vi "Continuous Pulse Train Test (IPD).vi"() -> ()   [LabVIEW 2015]
uses:
  Waveform VIs/Pulse Train VIs/Pulse Train Params.ctl
  Waveform VIs/Pulse Train VIs/Pulse Polarity.ctl
  Waveform VIs/Pulse Train VIs/PT-Continuous State.ctl
  <vilib>/sound2/lvsound2.llb/Sound Data Format.ctl
  <vilib>/sound2/lvsound2.llb/Sampling Mode.ctl
  <vilib>/sound2/lvsound2.llb/Sound Output Write (DBL).vi
panel:
  in  "IPD (cycles)":dbl(slide)=0.5 min=-0.5 max=0.5 scale=-0.5..0.5
  in  "stop":bool
  in  "Sound Format":T1={"sample rate (S/s)"=50000.0, "number of channels"=2, "bits per sample"=16}
  in  "Device ID":u32
  in  "Pulse Train Params":T2={"Pulse width (us)"=100.0, "Pulse rate (Hz)"=0.0, "Gap (ms)"=0.0, "Polarity"=enum."NEG-POS", "PT State"={"Template"=[], "Nperiod"=0, "Index"=0, "Pulse Rate (Hz)"=0.0, "Phase (cycles)"=0.0, "Noff"=0}, "Asynch"=FALSE}
  out "Graph":waveform(dbl)[](graph)
  in  "Buffer (ms)":dbl=100.0
  in  "Pulse Rate (Hz)":dbl(slide)=36.55555555555556 min=1.0 max=100.0 scale=1.0..100.0
  in  "Fs (Hz)":dbl=100000.0
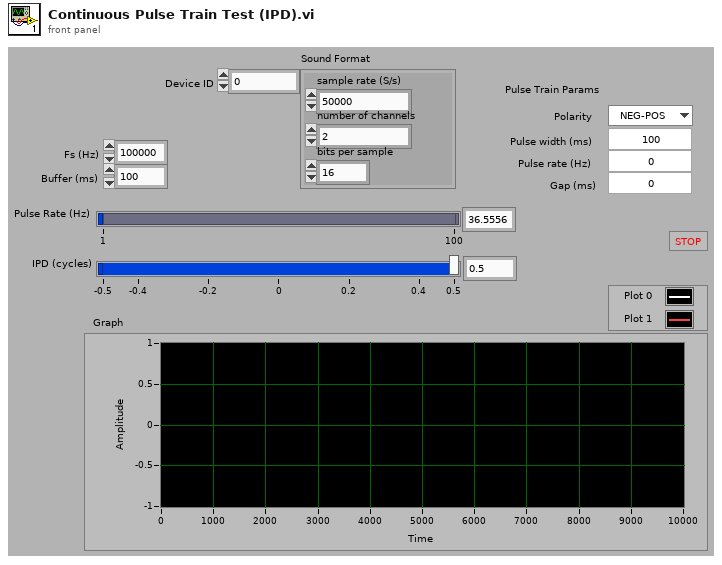
[diagram p1: front panel]
types:
  T1 = typedef "Sound Data Format.ctl" = cluster{"sample rate (S/s)":dbl, "number of channels":i32, "bits per sample":i32}
  T2 = typedef "Pulse Train Params.ctl" = cluster{"Pulse width (us)":dbl, "Pulse rate (Hz)":dbl, "Gap (ms)":dbl, "Polarity":T3, "PT State":T4, "Asynch":bool}
  T3 = typedef "Pulse Polarity.ctl" = enum16{"POS", "NEG", "POS-NEG", "NEG-POS"}
  T4 = typedef "PT-Continuous State.ctl" = cluster{"Template":dbl[], "Nperiod":i32, "Index":i32, "Pulse Rate (Hz)":dbl, "Phase (cycles)":dbl, "Noff":i32}
  T5 = typedef "Sampling Mode.ctl" = i32
  T6 = typedef "Sound Output Task ID.ctl" = u32
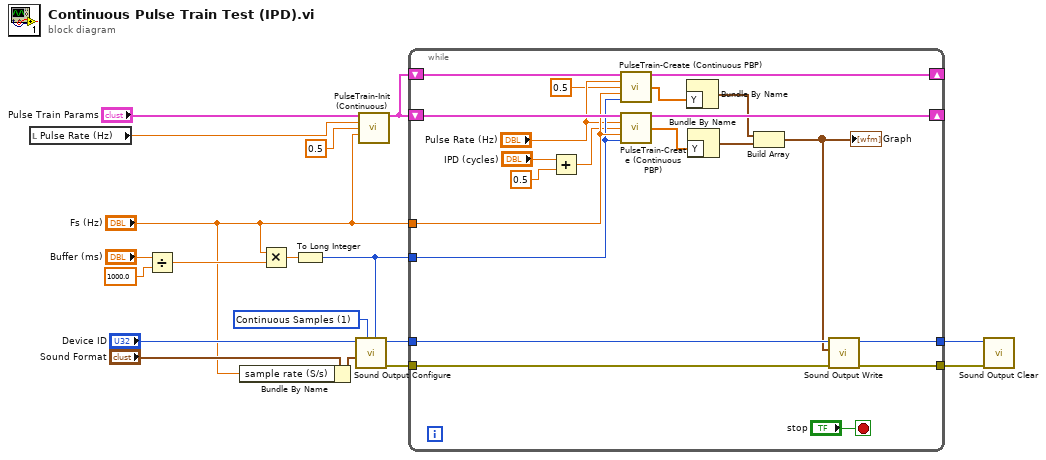
[diagram p0: block diagram]
diagram:
  w12 = T5 1 items=["Finite Samples", "Continuous Samples"] ("sample mode")
  n1 = local read "Pulse Rate (Hz)"() -> (w3:dbl)
  n2 = Divide(x="Buffer (ms)", y=1000.0) -> (x/y=w16:dbl)
  n3 = Bundle By Name(cluster="Sound Format", "sample rate (S/s)"="Fs (Hz)") -> (w10:T1)
  n4 = Multiply(x="Fs (Hz)", y=w16) -> (x*y=w15:dbl)
  n5 = To Long Integer(number=w15) -> (32bit integer=w9:i32)
  n6 = call <vilib>:"Sound Output Configure.vi"("number of samples/ch"=w9, "sample mode"=w12, "sound format"=w10, "device ID"="Device ID") -> ("error out"=w6:errorcluster, "task ID"=w7:T6)  [unwired: 6 in]
  n7 = call "PulseTrain-Init (Continuous).vi"("Pulse Train Params"="Pulse Train Params", "Start Pulse Rate (Hz)"=w3, "Start Phase (cycles)"=0.5, "Fs (Hz)"="Fs (Hz)") -> ("Initial State"=w1:T4)  [unwired: 10 in, 1 out]
  n8 = while {
    tunnel: w9 -> [w26]
    tunnel: "Fs (Hz)" -> [w27]
    shift-right: [w38] -> _
    shift-left: w1 -> [w39]
    tunnel: w7 -> [w35]
    tunnel: w6 -> [w36]
    tunnel: [w34] -> w5
    tunnel: [w33] -> w4
    shift-right: [w28] -> _
    shift-left: w1 -> [w29]
    stop <- "stop" stop-if-true
    n9 = Add(x="IPD (cycles)", y=0.5 ("Phase (cycles)")) -> (x+y=w20:dbl)
    n10 = call "PulseTrain-Create (Continuous PBP).vi"("State In"=w29, "Pulse Rate (Hz)"="Pulse Rate (Hz)", "Phase (cycles)"=0.5, "Fs (Hz)"=w27, "Npts"=w26) -> ("State Out"=w28:T4, "Buffer"=w23:dbl[])  [unwired: 8 in, 1 out]
    n11 = call "PulseTrain-Create (Continuous PBP).vi"("State In"=w39, "Pulse Rate (Hz)"="Pulse Rate (Hz)", "Phase (cycles)"=w20, "Fs (Hz)"=w27, "Npts"=w26) -> ("State Out"=w38:T4, "Buffer"=w32:dbl[])  [unwired: 8 in, 1 out]
    n12 = Bundle By Name("Y"=w23) -> (w22:waveform(dbl))  [unwired: 1 in]
    n13 = Bundle By Name("Y"=w32) -> (w30:waveform(dbl))  [unwired: 1 in]
    n14 = Build Array(w22, w30) -> (w21:waveform(dbl)[])
    "Graph" <- w21
    n15 = call-poly <vilib>:"Sound Output Write.vi"("error in (no error)"=w36, "data"=w21, "task ID"=w35) -> ("error out"=w33:errorcluster, "task ID out"=w34:T6)  [unwired: 7 in]
  }
  n16 = call <vilib>:"Sound Output Clear.vi"("error in (no error)"=w4, "task ID"=w5) -> ()  [unwired: 9 in, 1 out]
